vi "Destroy.vi"(8 "error in (no error)":errorcluster, 11 "Text In":refnum<class "Text.lvclass">) -> (0 "error out":errorcluster, 3 "Text Out":refnum<class "Text.lvclass">)   [LabVIEW 2015, in "Front Panel Publisher.lvlib" / "Text.lvclass"]
uses:
  Text.lvclass
  Object_class/Object.lvclass
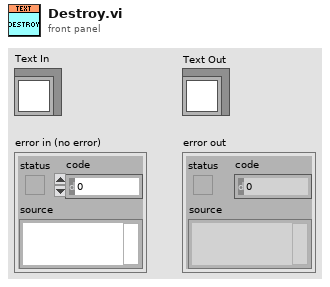
[diagram p1: front panel]
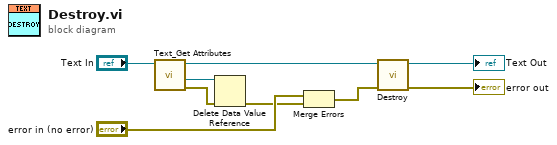
[diagram p0: block diagram]
diagram:
  n1 = call "Text_Get Attributes.vi"("Text In"="Text In") -> ("error out"=w8:errorcluster, "DataRef"=w7:refnum<data-value>, "Text Out"=w3:refnum<class "Text.lvclass">)  [unwired: 7 in, 1 out]
  n2 = Delete Data Value Reference(data value reference=w7, error in=w8) -> (error out=w5:errorcluster)  [unwired: 1 out]
  n3 = Merge Errors("error in (no error)", w5) -> (w4:errorcluster)
  n4 = call-parent "Destroy.vi"("error in (no error)"=w4, "Object In"=w3) -> ("error out"=→"error out":errorcluster, "Object Out"=→"Text Out":refnum<class "Text.lvclass">)  [unwired: 8 in]
